vi "禹山溶解氧校准.vi"() -> ()   [LabVIEW 2016, in "斯坦道多参数.lvlib"]
uses:
  <vilib>/Utility/miscctls.llb/LVPointTypeDef.ctl
  <vilib>/Analysis/NI_AALBase.lvlib
  <vilib>/Analysis/NI_AALPro.lvlib
  <vilib>/Utility/config.llb/NI_LVConfig.lvlib
panel:
  in  "盐度自动获取":bool
  in  "大气压补偿":dbl
  in  "盐度补偿":dbl
  out "DO %":dbl caption="饱和度值"
  out "第二点校准值":dbl
  out "第一点校准值":dbl
  out "最小值":sgl format="%.2g"
  out "最大值":sgl format="%.2g"
  in  "校准停止":bool
  in  "校准模式":enum16{"两点校准", "单点校准"}(ring)
  in  "标液2":dbl
  in  "标液1":dbl
  out "波形图表":sgl(graph) caption="历史曲线"
  out "温度测量值":dbl caption="温度"
  out "变异系数":dbl format="%.6g"
  out "standard deviation":dbl caption="标准差" format="%0.2f"
  out "mean":dbl caption="均值" format="%0.2f"
  out "提示":string
  in  "校准启动":bool
  out "DO mg/L":dbl caption="测试值"
  out "电极斜率":dbl
  out "电极零点":dbl
  # "溶解氧电极设定"
  # "℃"
  # "%"
  # "mg/L"
  # "kPa"
  # "请选择校准模式:"
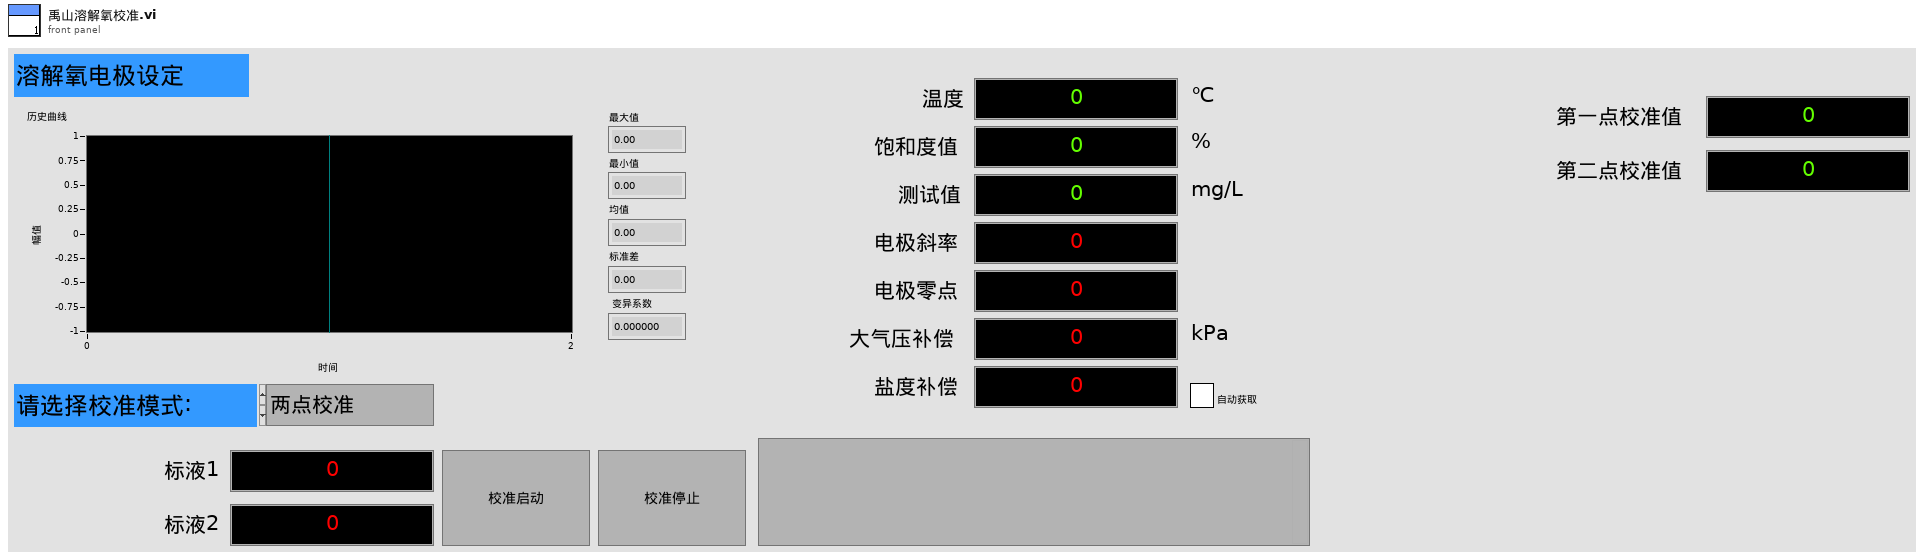
[diagram p1: front panel]
types:
  T1 = typedef "斯坦道多参数.lvlib/校准步骤.ctl" = enum16{"待机", "放置第一点标液", "第一点校准启动", "第一点校准写入", "第一点校准失败", "放置第二点标液", "第二点校准启动", "第二点校准写入", "第二点校准失败", "校准结果写入", "校准结束"}
  T2 = typedef "LVPointTypeDef.ctl" = cluster{"Horizontal":i16, "Vertical":i16}
  T3 = typedef "NI_LVConfig.lvlib/Config Data RefNum.ctl" = refnum<k1>
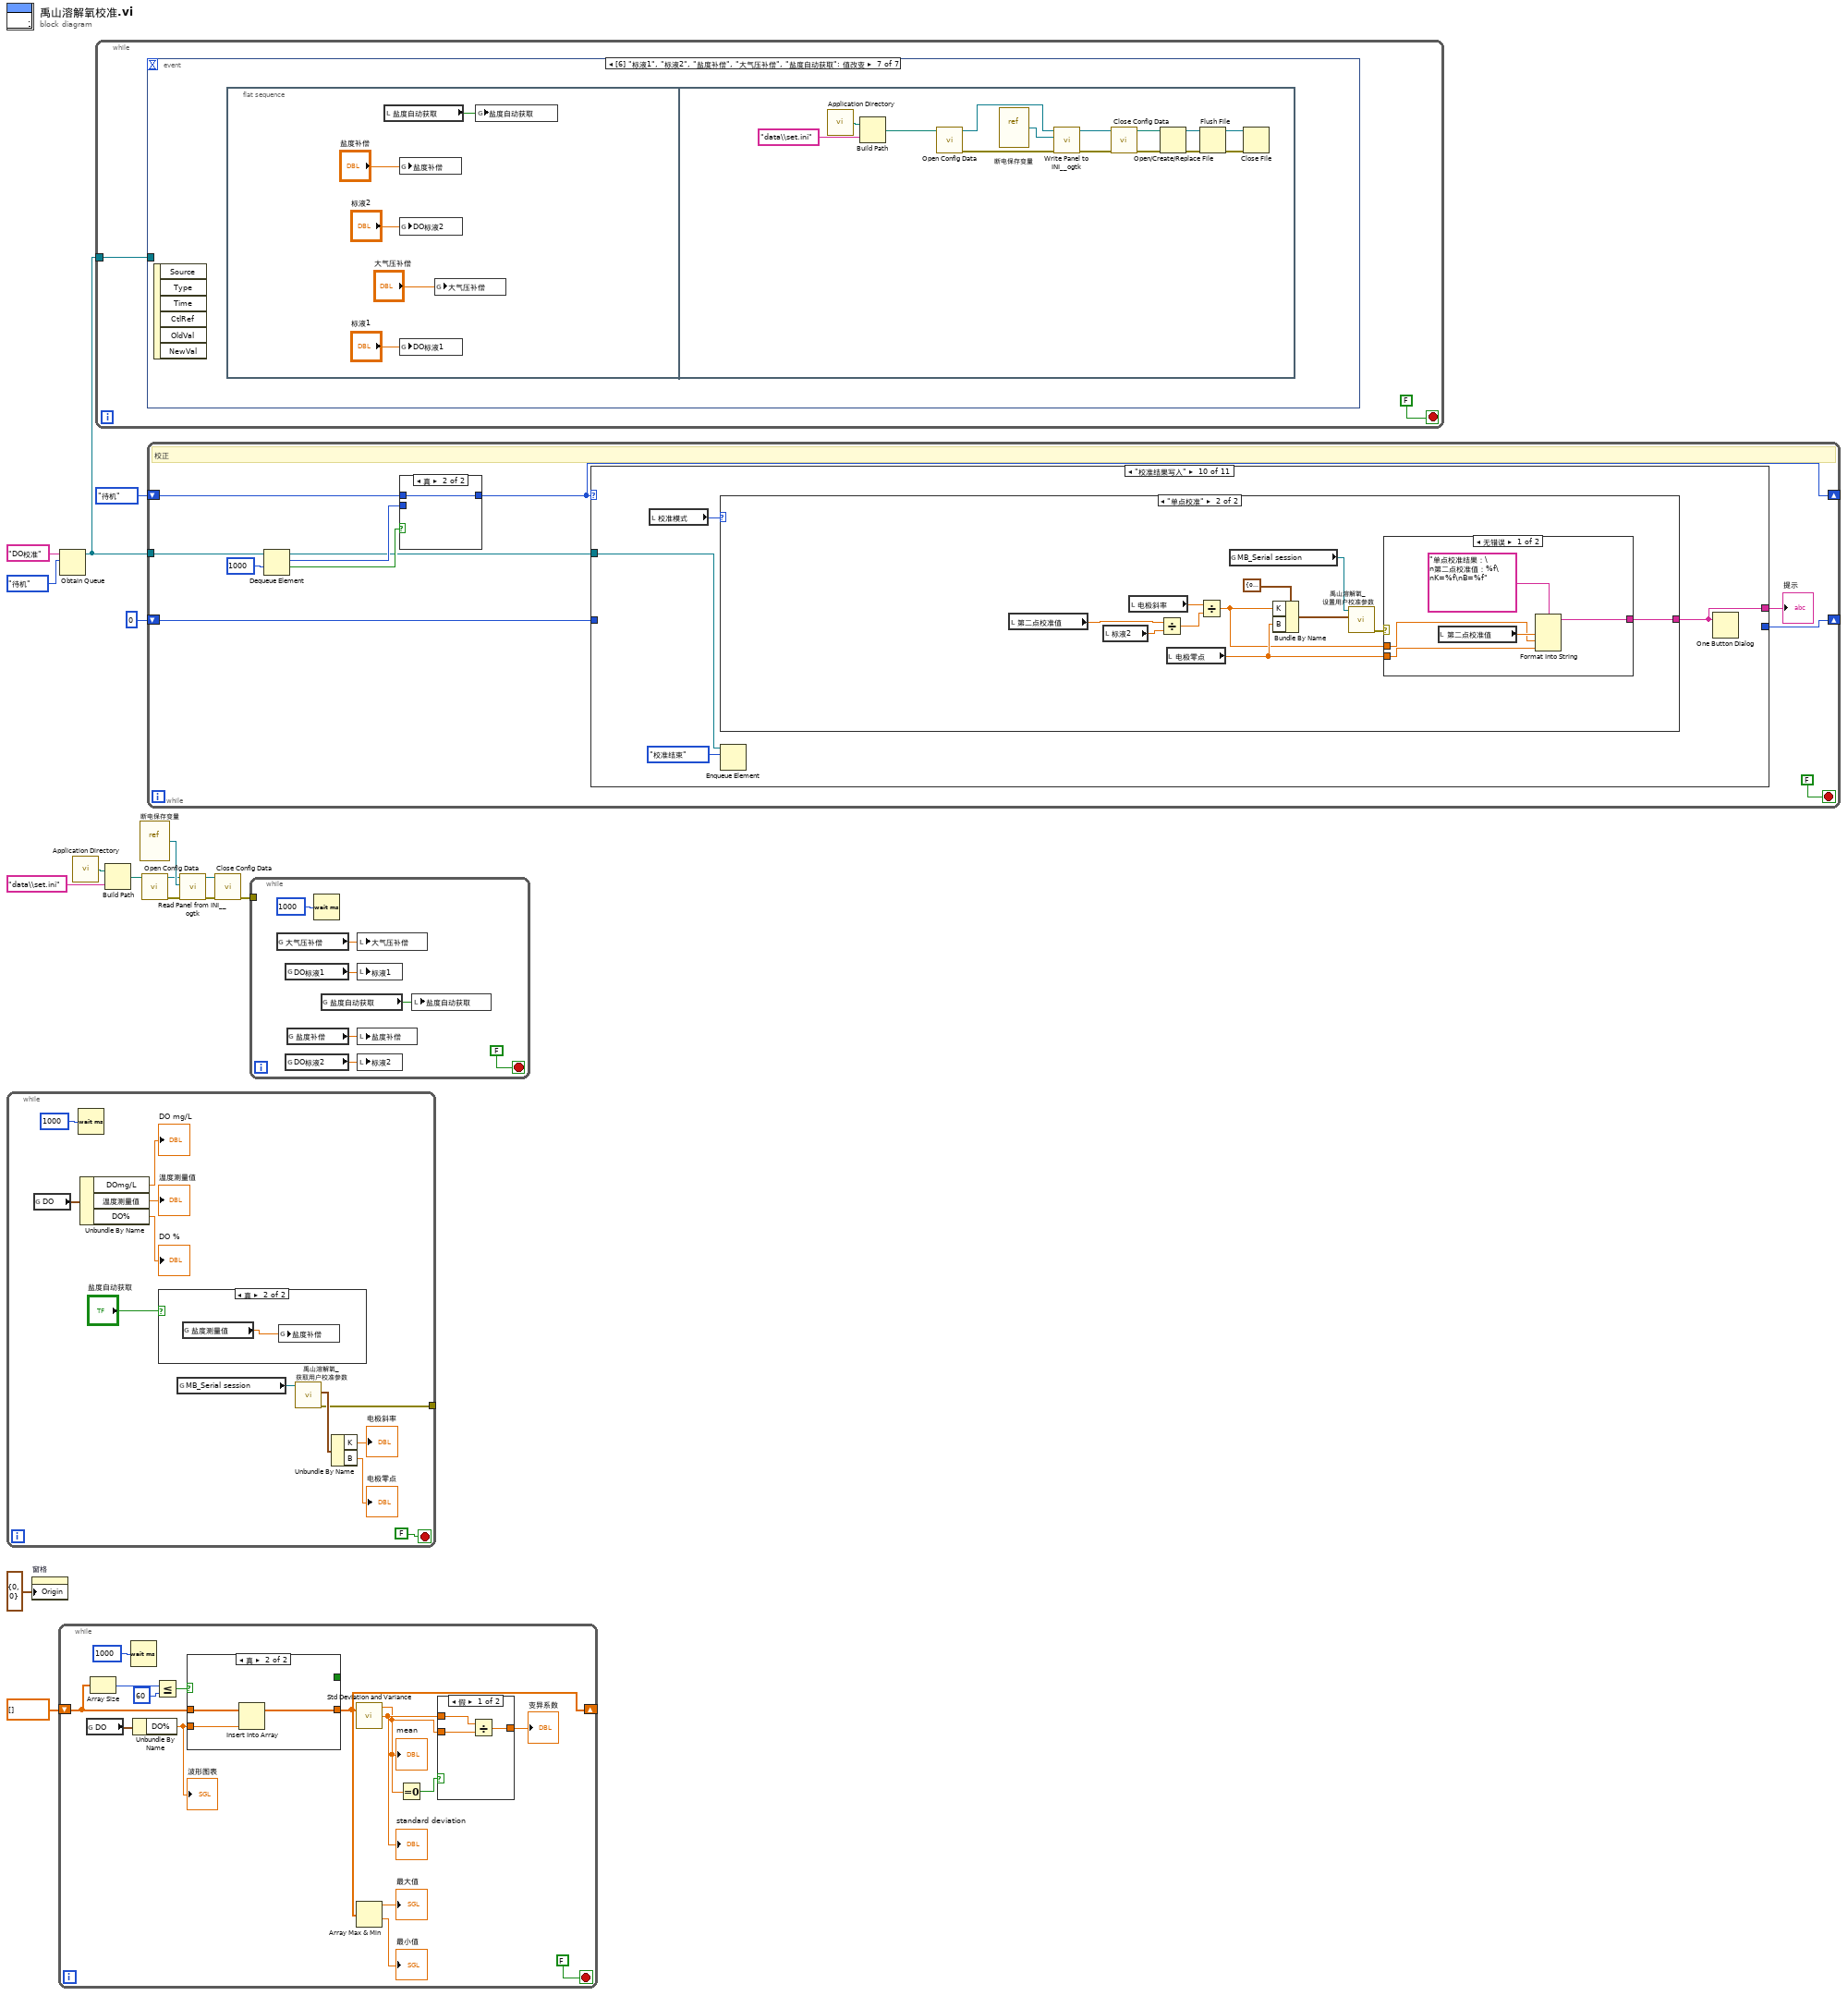
[diagram p0: block diagram]
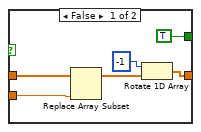
[diagram p3: hidden frame]
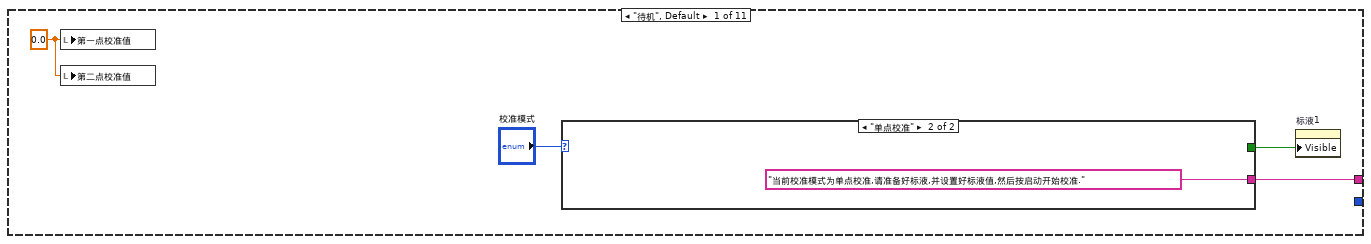
[diagram p5: hidden frame]
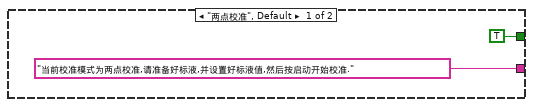
[diagram p6: hidden frame]
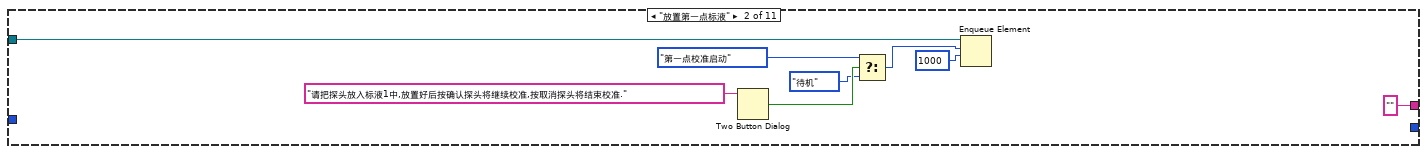
[diagram p7: hidden frame]
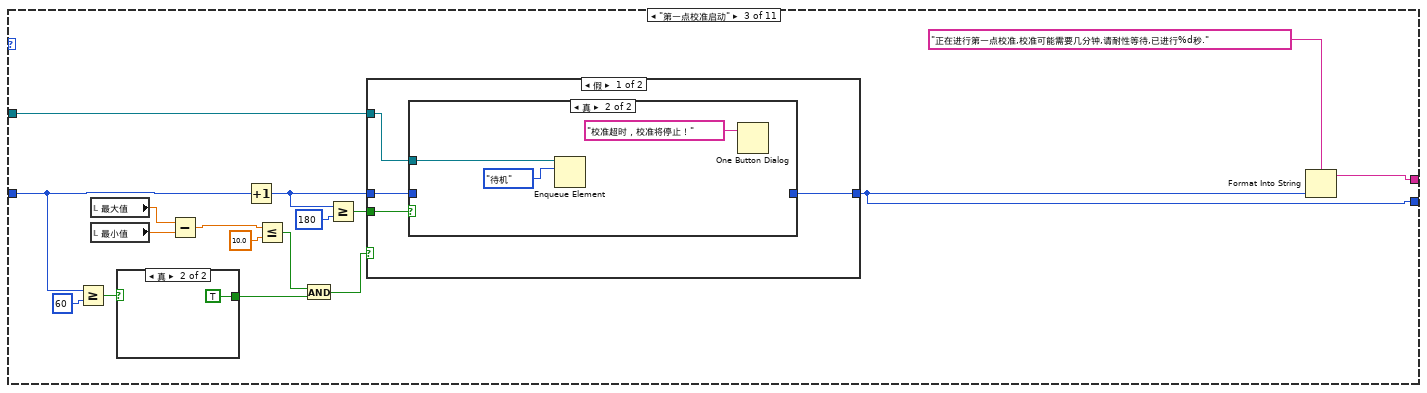
[diagram p8: hidden frame]
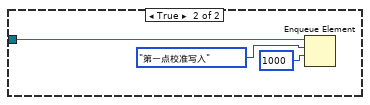
[diagram p10: hidden frame]
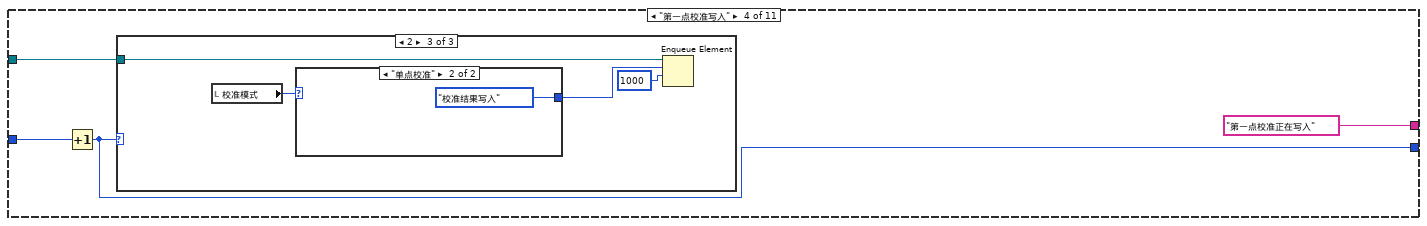
[diagram p12: hidden frame]
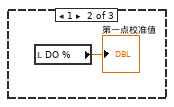
[diagram p14: hidden frame]
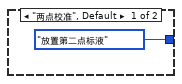
[diagram p15: hidden frame]
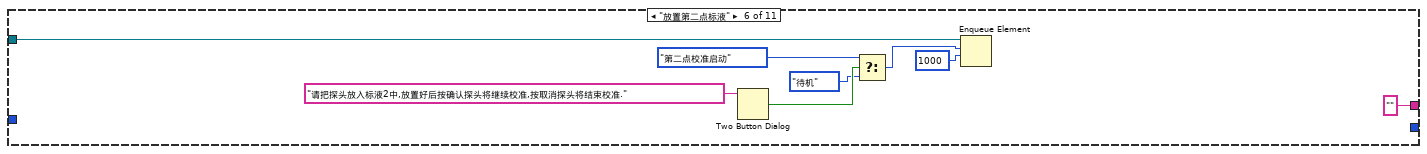
[diagram p17: hidden frame]
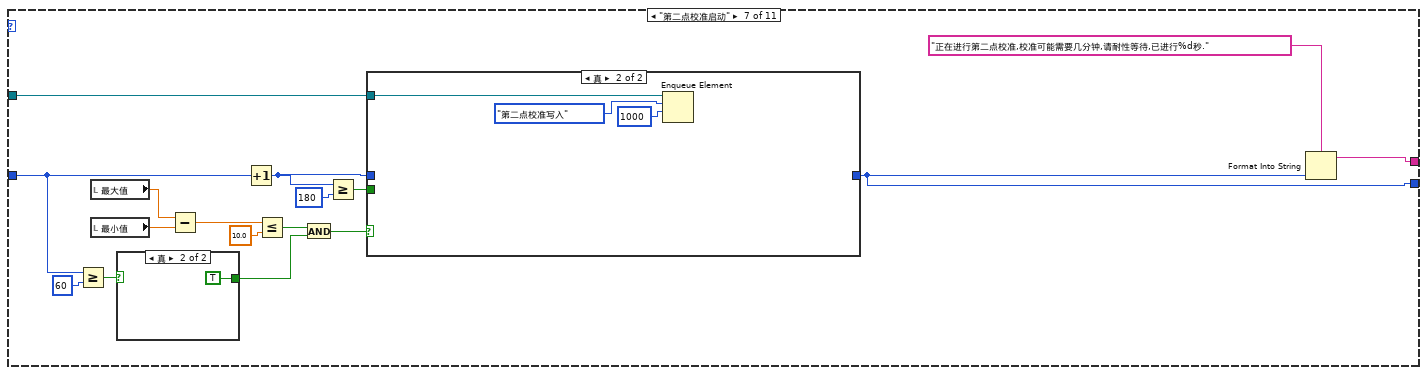
[diagram p18: hidden frame]
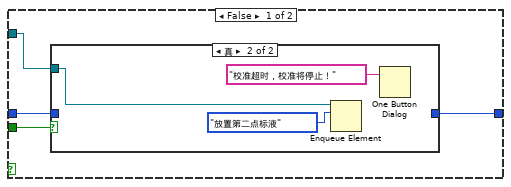
[diagram p19: hidden frame]
diagram:
  n1 = while {
    tunnel: [w23] -> _
    stop <- FALSE stop-if-true
    n2 = global read "禹山过程全局变量.vi" "DO"() -> (w20:cluster{"温度测量值":sgl, "DO%":sgl, "DOmg/L":sgl})
    n3 = Wait (ms)(milliseconds to wait=u32 1000 ("等待时间（毫秒）")) -> ()  [unwired: 1 out]
    n4 = Unbundle By Name(w20) -> ("DOmg/L"=→"DO mg/L":sgl, "温度测量值"=→"温度测量值":sgl, "DO%"=→"DO %":sgl)
    n5 = case shown="真" "盐度自动获取" {
      frame False {
      }
      frame True {
        n6 = global read "国弘过程全局变量.vi" "盐度测量值"() -> (w29:sgl)
        n7 = global write "断电保存变量.vi" "盐度补偿"(w29) -> ()
      }
    }
    n8 = global read "多参数全局变量.vi" "MB_Serial session"() -> (w19:refnum<class "MB_Master_Serial.lvclass">)
    n9 = call "禹山溶解氧_获取用户校准参数.vi"("MB_Serial session in"=w19) -> ("error out"=w23:errorcluster, "输出值"=w26:cluster{"K":sgl, "B":sgl})  [unwired: 8 in, 1 out]
    n10 = Unbundle By Name(w26) -> ("K"=→"电极斜率":sgl, "B"=→"电极零点":sgl)
  }
  n11 = property on="窗格" class="Pane"("Origin"=T2 {"Horizontal"=0, "Vertical"=0} ("原点")) -> ()  [unwired: 2 in, 2 out]
  n12 = while {
    shift-right: [w32] -> _
    shift-left: sgl[] [] -> [w40]
    stop <- FALSE stop-if-true
    n13 = global read "禹山过程全局变量.vi" "DO"() -> (w34:cluster{"温度测量值":sgl, "DO%":sgl, "DOmg/L":sgl})
    n14 = Array Size(array=w40) -> (size(s)=w42:i32)
    n15 = Wait (ms)(milliseconds to wait=u32 1000 ("等待时间（毫秒）")) -> ()  [unwired: 1 out]
    n16 = Unbundle By Name(w34) -> ("DO%"=w33:sgl)
    "波形图表" <- w33
    n17 = Less Or Equal?(x=w42, y=60) -> (x <= y?=w41:bool)
    n18 = case shown="真" w41 {
      tunnel: w40 -> [w53 w56]
      tunnel: w33 -> [w51 w55]
      tunnel: [w49 w54] -> w32
      tunnel: [TRUE _] -> _
      frame False {
        n19 = Replace Array Subset(array=w53, new element=w51) -> (w52:sgl[])  [unwired: 1 in]
        n20 = Rotate 1D Array(1:w52, 2:-1 ("n")) -> (0:w49:sgl[])
      }
      frame True {
        n21 = Insert Into Array(array=w56, new element=w55) -> (w54:sgl[])  [unwired: 1 in]
      }
    }
    n22 = call <vilib>:"Std Deviation and Variance.vi"("X"=w32) -> ("mean"=w35:dbl, "standard deviation"=w36:dbl)  [unwired: 1 in, 1 out]
    "standard deviation" <- w36
    "mean" <- w35
    n23 = Array Max & Min(array=w32) -> (max value=→"最大值":sgl, min value=→"最小值":sgl)  [unwired: 2 out]
    n24 = Equal To 0?(x=w35) -> (x = 0?=w39:bool)
    n25 = case shown="假" w39 {
      tunnel: w36 -> [w47 _]
      tunnel: [w46 _] -> w38
      tunnel: w35 -> [w45 _]
      frame False {
        n26 = Divide(x=w47, y=w45) -> (x/y=w46:dbl)
      }
      frame True {
      }
    }
    "变异系数" <- w38
  }
  n27 = Obtain Queue(name (unnamed)="DO校准" ("名称（未命名）"), element data type=校准步骤."待机" ("枚举")) -> (queue out=w10:refnum<queue>)  [unwired: 3 in, 2 out]
  n28 = call <vilib>:"Application Directory.vi"() -> ("Application Directory"=w6:path)
  n29 = while {
    tunnel: w10 -> [w57]
    stop <- FALSE stop-if-true
    n30 = event shown="[6] \"标液1\", \"标液2\", \"盐度补偿\", \"大气压补偿\", \"盐度自动获取\": 值改变" {
      selector: _ -> [_ _ _ _ _ _ _]
      dyn-events: _ -> [_ _ _ _ _ _ _]
      timeout: _ -> [_ _ _ _ _ _ _]
      tunnel: w57 -> [_ w61 w67 _ _ _ _]
      event Timeout {
        n31 = event-data() -> ()  [unwired: 1 in, 3 out]
      }
      event "校准启动": Value Change {
        n32 = event-data() -> ()  [unwired: 1 in, 6 out]
        n33 = local read "校准模式"() -> (w60:enum16{"两点校准", "单点校准"})
        n34 = case shown="\"两点校准\", 默认" w60 {
          tunnel: [校准步骤."放置第一点标液" ("元素") 校准步骤."放置第二点标液" ("元素")] -> w59
          frame "两点校准", Default {
          }
          frame "单点校准" {
          }
        }
        n35 = Enqueue Element(queue=w61, element=w59) -> ()  [unwired: 2 in, 3 out]
      }
      event "校准停止": Value Change {
        n36 = event-data() -> ()  [unwired: 1 in, 6 out]
        n37 = Flush Queue(queue=w67) -> (queue out=w64:refnum<queue>)  [unwired: 1 in, 2 out]
        n38 = Enqueue Element(queue=w64, element=校准步骤."待机" ("元素"), timeout in ms (-1)=1000 ("超时毫秒(-1)")) -> ()  [unwired: 1 in, 3 out]
      }
      event "电极零点", "电极斜率", "标液1", "标液2", "大气压补偿": Mouse Down {
        n39 = event-data() -> ("CtlRef"=w68:refnum<vi>)  [unwired: 1 in, 7 out]
        n40 = property class="DigNum (严格)"(reference=w68) -> (reference out=w69:refnum<vi>, "Value"=w70:dbl)  [unwired: 1 in, 1 out]
        n41 = call "数字键盘.vi"("OldNumber"=w70) -> ("NewNumber"=w71:sgl)
        n42 = property class="DigNum (严格)"(reference=w69, "Val(Sgnl)"=w71) -> ()  [unwired: 1 in, 2 out]
      }
      event "盐度补偿": Mouse Down {
        n43 = event-data() -> ("CtlRef"=w73:refnum<vi>)  [unwired: 1 in, 7 out]
        n44 = local read "盐度自动获取"() -> (w72:bool)
        n45 = case shown="假" w72 {
          tunnel: w73 -> [w74 _]
          frame False {
            n46 = property class="DigNum (严格)"(reference=w74) -> (reference out=w75:refnum<vi>, "Value"=w76:dbl)  [unwired: 1 in, 1 out]
            n47 = call "数字键盘.vi"("OldNumber"=w76) -> ("NewNumber"=w77:sgl)
            n48 = property class="DigNum (严格)"(reference=w75, "Val(Sgnl)"=w77) -> ()  [unwired: 1 in, 2 out]
          }
          frame True {
          }
        }
      }
      event "电极零点", "电极斜率": Value Change {
        n49 = event-data() -> ()  [unwired: 1 in, 6 out]
        n50 = local read "电极斜率"() -> (w80:dbl)
        n51 = local read "电极零点"() -> (w79:dbl)
        n52 = global read "多参数全局变量.vi" "MB_Serial session"() -> (w78:refnum<class "MB_Master_Serial.lvclass">)
        n53 = Bundle By Name(cluster=cluster{"K":sgl, "B":sgl} {"K"=0.0, "B"=0.0} ("用户校准参数"), "K"=w80, "B"=w79) -> (w81:cluster{"K":sgl, "B":sgl})
        n54 = call "禹山溶解氧_设置用户校准参数.vi"("用户校准参数"=w81, "MB_Serial session in"=w78) -> ()  [unwired: 8 in, 2 out]
      }
      event "标液1", "标液2", "盐度补偿", "大气压补偿", "盐度自动获取": Value Change {
        n55 = event-data() -> ()  [unwired: 1 in, 6 out]
        n56 = flat-sequence {
          frame #0 {
            n57 = local read "盐度自动获取"() -> (w83:bool)
            n58 = global write "断电保存变量.vi" "盐度补偿"("盐度补偿") -> ()
            n59 = global write "断电保存变量.vi" "DO标液2"("标液2") -> ()
            n60 = global write "断电保存变量.vi" "DO标液1"("标液1") -> ()
            n61 = global write "断电保存变量.vi" "大气压补偿"("大气压补偿") -> ()
            n62 = global write "断电保存变量.vi" "盐度自动获取"(w83) -> ()
          }
          frame #1 {
            n63 = call <vilib>:"Application Directory.vi"() -> ("Application Directory"=w97:path)
            n64 = Build Path(base path=w97, name or relative path="data\\set.ini" ("名称或相对路径")) -> (appended path=w96:path)
            n65 = call <vilib>:"Open Config Data.vi"("configuration file path"=w96) -> ("error out"=w100:errorcluster, "refnum"=w101:T3)  [unwired: 8 in, 1 out]
            n66 = vi-ref "断电保存变量.vi"() -> (w94:refnum<vi>)
            n67 = call <userlib>:"Write Panel to INI__ogtk.vi"("error in (no error)"=w100, "VI ref"=w94, "refnum"=w101) -> ("error out"=w98:errorcluster, "refnum out"=w99:T3)  [unwired: 7 in]
            n68 = call <vilib>:"Close Config Data.vi"("error in (no error)"=w98, "refnum"=w99) -> ("error out"=w90:errorcluster, "file path"=w91:path)  [unwired: 8 in]
            n69 = Open/Create/Replace File(file path (use dialog)=w91, error in=w90) -> (refnum out=w92:refnum<file>, error out=w93:errorcluster)  [unwired: 4 in, 1 out]
            n70 = Flush File(refnum=w92, error in=w93) -> (refnum out=w88:refnum<file>, error out=w89:errorcluster)
            n71 = Close File(refnum=w88, error in=w89) -> ()  [unwired: 2 out]
          }
        }
      }
    }
  }
  n72 = Build Path(base path=w6, name or relative path="data\\set.ini" ("名称或相对路径")) -> (appended path=w7:path)
  n73 = vi-ref "断电保存变量.vi"() -> (w9:refnum<vi>)
  n74 = call <vilib>:"Open Config Data.vi"("configuration file path"=w7) -> ("error out"=w3:errorcluster, "refnum"=w2:T3)  [unwired: 8 in, 1 out]
  n75 = while "While循环" {
    shift-right: [w103] -> _
    shift-left: 校准步骤."待机" ("枚举") -> [w104]
    shift-right: [w110] -> _
    shift-left: 0 -> [w111]
    tunnel: w10 -> [w108]
    stop <- FALSE stop-if-true
    # "校正"
    n76 = Dequeue Element(queue=w108, timeout in ms (-1)=1000 ("超时毫秒(-1)")) -> (queue out=w102:refnum<queue>, element=w105:T1, timed out?=w106:bool)  [unwired: 1 in, 1 out]
    n77 = case shown="真" w106 {
      tunnel: w105 -> [w113 _]
      tunnel: [w113 w114] -> w103
      tunnel: w104 -> [_ w114]
      frame False {
      }
      frame True {
      }
    }
    n78 = case shown="\"校准结果写入\"" w103 {
      tunnel: [w118 "" ("提示") w145 "第一点校准正在写入" ("提示") _ "" ("提示") w193 "第二点校准正在写入" ("提示") _ w218 w265] -> w109
      tunnel: w111 -> [_ _ w139 w161 _ _ w187 w209 _ _ _]
      tunnel: [_ _ w130 w160 _ _ w178 w208 _ _ _] -> w110
      tunnel: w102 -> [_ w128 w133 w159 _ w176 w181 w207 _ w217 _]
      frame "待机", Default {
        w115 = 0.0 ("第一点校准值")
        n79 = local write "第一点校准值"(w115) -> ()
        n80 = local write "第二点校准值"(w115) -> ()
        n81 = case shown="\"单点校准\"" "校准模式" {
          tunnel: ["当前校准模式为两点校准,请准备好标液,并设置好标液值,然后按启动开始校准." ("提示") "当前校准模式为单点校准,请准备好标液,并设置好标液值,然后按启动开始校准." ("提示")] -> w118
          tunnel: [TRUE ("可见") _] -> w116
          frame "两点校准", Default {
          }
          frame "单点校准" {
          }
        }
        n82 = property on="标液1" class="DigNum (严格)"("Visible"=w116) -> ()  [unwired: 2 in, 2 out]
      }
      frame "放置第一点标液" {
        n83 = Two Button Dialog(message="请把探头放入标液1中,放置好后按确认探头将继续校准,按取消探头将结束校准." ("消息")) -> (T button?=w126:bool)  [unwired: 2 in]
        n84 = Select(t=校准步骤."第一点校准启动" ("元素"), s=w126, f=校准步骤."待机" ("元素")) -> (s? t:f=w123:T1)
        n85 = Enqueue Element(queue=w128, element=w123, timeout in ms (-1)=1000 ("超时毫秒(-1)")) -> ()  [unwired: 1 in, 3 out]
      }
      frame "第一点校准启动" {
        n86 = Greater Or Equal?(x=w139, y=60) -> (x >= y?=w140:bool)
        n87 = local read "最大值"() -> (w136:sgl)
        n88 = local read "最小值"() -> (w137:sgl)
        n89 = case shown="真" w140 {
          tunnel: [_ TRUE] -> w138
          frame False {
          }
          frame True {
          }
        }
        n90 = Subtract(x=w136, y=w137) -> (x-y=w135:sgl)
        n91 = Increment(x=w139) -> (x+1=w131:i32)
        n92 = Less Or Equal?(x=w135, y=10.0) -> (x <= y?=w143:bool)
        n93 = And(x=w143, y=w138) -> (x .and. y?=w134:bool)
        n94 = Greater Or Equal?(x=w131, y=180) -> (x >= y?=w132:bool)
        n95 = case shown="假" w134 {
          tunnel: w133 -> [w149 w157]
          tunnel: w132 -> [w150 _]
          tunnel: w131 -> [w148 _]
          tunnel: [w147 _] -> w130
          frame False {
            n96 = case shown="真" w150 {
              tunnel: w149 -> [_ w154]
              tunnel: w148 -> [w151 _]
              tunnel: [w151 _] -> w147
              frame False {
              }
              frame True {
                n97 = Enqueue Element(queue=w154, element=校准步骤."待机" ("元素")) -> ()  [unwired: 2 in, 3 out]
                n98 = One Button Dialog(message="校准超时，校准将停止！" ("消息")) -> ()  [unwired: 1 in, 1 out]
              }
            }
          }
          frame True {
            n99 = Enqueue Element(queue=w157, element=校准步骤."第一点校准写入" ("元素"), timeout in ms (-1)=1000 ("超时毫秒(-1)")) -> ()  [unwired: 1 in, 3 out]
          }
        }
        n100 = Format Into String(format string="正在进行第一点校准,校准可能需要几分钟,请耐性等待,已进行%d秒." ("格式字符串"), w130) -> (resulting string=w145:string)  [unwired: 2 in, 1 out]
      }
      frame "第一点校准写入" {
        n101 = Increment(x=w161) -> (x+1=w160:i32)
        n102 = case shown="2" w160 {
          tunnel: w159 -> [_ _ w167]
          frame 0, Default {
          }
          frame 1 {
            n103 = local read "DO %"() -> (→"第一点校准值":dbl)
          }
          frame 2 {
            n104 = local read "校准模式"() -> (w166:enum16{"两点校准", "单点校准"})
            n105 = case shown="\"单点校准\"" w166 {
              tunnel: [校准步骤."放置第二点标液" ("元素") 校准步骤."校准结果写入" ("元素")] -> w165
              frame "两点校准", Default {
              }
              frame "单点校准" {
              }
            }
            n106 = Enqueue Element(queue=w167, element=w165, timeout in ms (-1)=1000 ("超时毫秒(-1)")) -> ()  [unwired: 1 in, 3 out]
          }
        }
      }
      frame "第一点校准失败" {
      }
      frame "放置第二点标液" {
        n107 = Two Button Dialog(message="请把探头放入标液2中,放置好后按确认探头将继续校准,按取消探头将结束校准." ("消息")) -> (T button?=w174:bool)  [unwired: 2 in]
        n108 = Select(t=校准步骤."第二点校准启动" ("元素"), s=w174, f=校准步骤."待机" ("元素")) -> (s? t:f=w171:T1)
        n109 = Enqueue Element(queue=w176, element=w171, timeout in ms (-1)=1000 ("超时毫秒(-1)")) -> ()  [unwired: 1 in, 3 out]
      }
      frame "第二点校准启动" {
        n110 = Greater Or Equal?(x=w187, y=60) -> (x >= y?=w188:bool)
        n111 = local read "最大值"() -> (w184:sgl)
        n112 = local read "最小值"() -> (w185:sgl)
        n113 = case shown="真" w188 {
          tunnel: [_ TRUE] -> w186
          frame False {
          }
          frame True {
          }
        }
        n114 = Subtract(x=w184, y=w185) -> (x-y=w183:sgl)
        n115 = Increment(x=w187) -> (x+1=w179:i32)
        n116 = Less Or Equal?(x=w183, y=10.0) -> (x <= y?=w191:bool)
        n117 = And(x=w191, y=w186) -> (x .and. y?=w182:bool)
        n118 = Greater Or Equal?(x=w179, y=180) -> (x >= y?=w180:bool)
        n119 = case shown="真" w182 {
          tunnel: w181 -> [w197 w205]
          tunnel: w180 -> [w198 _]
          tunnel: w179 -> [w196 _]
          tunnel: [w195 _] -> w178
          frame False {
            n120 = case shown="真" w198 {
              tunnel: w197 -> [_ w202]
              tunnel: w196 -> [w199 _]
              tunnel: [w199 _] -> w195
              frame False {
              }
              frame True {
                n121 = Enqueue Element(queue=w202, element=校准步骤."放置第二点标液" ("元素")) -> ()  [unwired: 2 in, 3 out]
                n122 = One Button Dialog(message="校准超时，校准将停止！" ("消息")) -> ()  [unwired: 1 in, 1 out]
              }
            }
          }
          frame True {
            n123 = Enqueue Element(queue=w205, element=校准步骤."第二点校准写入" ("元素"), timeout in ms (-1)=1000 ("超时毫秒(-1)")) -> ()  [unwired: 1 in, 3 out]
          }
        }
        n124 = Format Into String(format string="正在进行第二点校准,校准可能需要几分钟,请耐性等待,已进行%d秒." ("格式字符串"), w178) -> (resulting string=w193:string)  [unwired: 2 in, 1 out]
      }
      frame "第二点校准写入" {
        n125 = Increment(x=w209) -> (x+1=w208:i32)
        n126 = case shown="1" w208 {
          tunnel: w207 -> [_ _ w214]
          frame 0, Default {
          }
          frame 1 {
            n127 = local read "DO %"() -> (→"第二点校准值":dbl)
          }
          frame 2 {
            n128 = Enqueue Element(queue=w214, element=校准步骤."校准结果写入" ("元素"), timeout in ms (-1)=1000 ("超时毫秒(-1)")) -> ()  [unwired: 1 in, 3 out]
          }
        }
      }
      frame "第二点校准失败" {
      }
      frame "校准结果写入" {
        n129 = local read "校准模式"() -> (w215:enum16{"两点校准", "单点校准"})
        n130 = case shown="\"单点校准\"" w215 {
          tunnel: [w228 w254] -> w218
          frame "两点校准", Default {
            n131 = local read "第一点校准值"() -> (w239:dbl)
            n132 = local read "第二点校准值"() -> (w238:dbl)
            n133 = local read "标液1"() -> (w236:dbl)
            n134 = local read "标液2"() -> (w235:dbl)
            n135 = Insert Into Array(array=dbl[] [] ("Weight"), new element #1=w236, new element #2=w235) -> (w234:dbl[])  [unwired: 1 in]
            n136 = Insert Into Array(array=dbl[] [] ("Weight"), new element #1=w239, new element #2=w238) -> (w233:dbl[])  [unwired: 1 in]
            n137 = call <vilib>:"Linear Fit.vi"("Y"=w234, "X"=w233) -> ("slope"=w227:dbl, "intercept"=w224:dbl)  [unwired: 9 in, 3 out]
            n138 = local read "电极斜率"() -> (w225:dbl)
            n139 = Divide(x=w224, y=100.0) -> (x/y=w220:dbl)
            n140 = local read "电极零点"() -> (w222:dbl)
            n141 = Multiply(x=w225, y=w220) -> (x*y=w223:dbl)
            n142 = Multiply(x=w227, y=w225) -> (x*y=w226:dbl)
            n143 = Add(x=w223, y=w222) -> (x+y=w221:dbl)
            n144 = global read "多参数全局变量.vi" "MB_Serial session"() -> (w232:refnum<class "MB_Master_Serial.lvclass">)
            n145 = Bundle By Name(cluster=cluster{"K":sgl, "B":sgl} {"K"=0.0, "B"=0.0} ("用户校准参数"), "K"=w226, "B"=w221) -> (w231:cluster{"K":sgl, "B":sgl})
            n146 = call "禹山溶解氧_设置用户校准参数.vi"("用户校准参数"=w231, "MB_Serial session in"=w232) -> ("error out"=w229:errorcluster)  [unwired: 8 in, 1 out]
            n147 = case shown="无错误" w229 {
              tunnel: w226 -> [w243 _]
              tunnel: w221 -> [w242 _]
              tunnel: [w241 "校准失败"] -> w228
              frame No Error {
                n148 = local read "第一点校准值"() -> (w245:dbl)
                n149 = local read "第二点校准值"() -> (w246:dbl)
                n150 = Format Into String(format string="两点校准结果：\n第一点校准值：%f\n第二点校准值：%f\nK=%f\nB=%f" ("提示"), w245, w246, w243, w242) -> (resulting string=w241:string)  [unwired: 2 in, 1 out]
              }
              frame Error {
              }
            }
          }
          frame "单点校准" {
            n151 = local read "第二点校准值"() -> (w252:dbl)
            n152 = local read "标液2"() -> (w251:dbl)
            n153 = local read "电极斜率"() -> (w249:dbl)
            n154 = Divide(x=w252, y=w251) -> (x/y=w248:dbl)
            n155 = local read "电极零点"() -> (w253:dbl)
            n156 = Divide(x=w249, y=w248) -> (x/y=w250:dbl)
            n157 = global read "多参数全局变量.vi" "MB_Serial session"() -> (w258:refnum<class "MB_Master_Serial.lvclass">)
            n158 = Bundle By Name(cluster=cluster{"K":sgl, "B":sgl} {"K"=0.0, "B"=0.0} ("用户校准参数"), "K"=w250, "B"=w253) -> (w257:cluster{"K":sgl, "B":sgl})
            n159 = call "禹山溶解氧_设置用户校准参数.vi"("用户校准参数"=w257, "MB_Serial session in"=w258) -> ("error out"=w255:errorcluster)  [unwired: 8 in, 1 out]
            n160 = case shown="无错误" w255 {
              tunnel: w250 -> [w261 _]
              tunnel: w253 -> [w260 _]
              tunnel: [w259 "校准失败"] -> w254
              frame No Error {
                n161 = local read "第二点校准值"() -> (w263:dbl)
                n162 = Format Into String(format string="单点校准结果：\n第二点校准值：%f\nK=%f\nB=%f" ("提示"), w263, w261, w260) -> (resulting string=w259:string)  [unwired: 2 in, 1 out]
              }
              frame Error {
              }
            }
          }
        }
        n163 = Enqueue Element(queue=w217, element=校准步骤."校准结束" ("元素")) -> ()  [unwired: 2 in, 3 out]
        n164 = One Button Dialog(message=w218) -> ()  [unwired: 1 in, 1 out]
      }
      frame "校准结束" {
        n165 = local read "提示"() -> (w265:string)
      }
    }
    "提示" <- w109
  }
  n166 = call <userlib>:"Read Panel from INI__ogtk.vi"("error in (no error)"=w3, "VI ref"=w9, "refnum"=w2) -> ("error out"=w5:errorcluster, "refnum out"=w4:T3)  [unwired: 7 in]
  n167 = call <vilib>:"Close Config Data.vi"("error in (no error)"=w5, "refnum"=w4) -> ("error out"=w1:errorcluster)  [unwired: 8 in, 1 out]
  n168 = while {
    tunnel: w1 -> [_]
    stop <- FALSE stop-if-true
    n169 = global read "断电保存变量.vi" "大气压补偿"() -> (w268:dbl)
    n170 = global read "断电保存变量.vi" "DO标液1"() -> (w270:dbl)
    n171 = global read "断电保存变量.vi" "DO标液2"() -> (w269:dbl)
    n172 = global read "断电保存变量.vi" "盐度补偿"() -> (w266:dbl)
    n173 = Wait (ms)(milliseconds to wait=u32 1000 ("等待时间（毫秒）")) -> ()  [unwired: 1 out]
    n174 = global read "断电保存变量.vi" "盐度自动获取"() -> (w267:bool)
    n175 = local write "大气压补偿"(w268) -> ()
    n176 = local write "标液1"(w270) -> ()
    n177 = local write "盐度补偿"(w266) -> ()
    n178 = local write "标液2"(w269) -> ()
    n179 = local write "盐度自动获取"(w267) -> ()
  }
